vi "RH200 READ FILE.vi"() -> ()   [LabVIEW 2014]
uses:
  <vilib>/Utility/file.llb/Write To Spreadsheet File (string).vi
  <vilib>/DAQmx/write.llb/DAQmx Write (Analog DBL 1Chan 1Samp).vi
  <vilib>/DAQmx/write.llb/DAQmx Write (Digital Bool 1Line 1Point).vi
  <vilib>/DAQmx/read.llb/DAQmx Read (Analog DBL 1Chan 1Samp).vi
panel:
  in  "RH file":path
  out "Data file":path
  in  "Delay (s)":dbl=2.0 caption="Wet MFC (V)" format="%#_13g"
  in  "Log data":bool
  out "Saving data":bool
  in  "stop":bool
  out "Waveform Chart":cluster{"RH Setpoint":dbl, "RH":dbl}(graph)
  in  "Temp":dbl=25.0 caption="Temp (C)" format="%#_13g"
  # "REBOOT RH GENERATOR BETWEEN USES TO RESET CONNECTION TO PC"
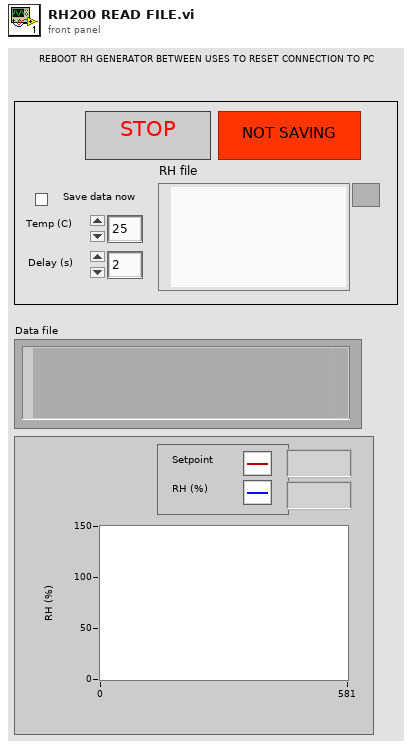
[diagram p1: front panel]
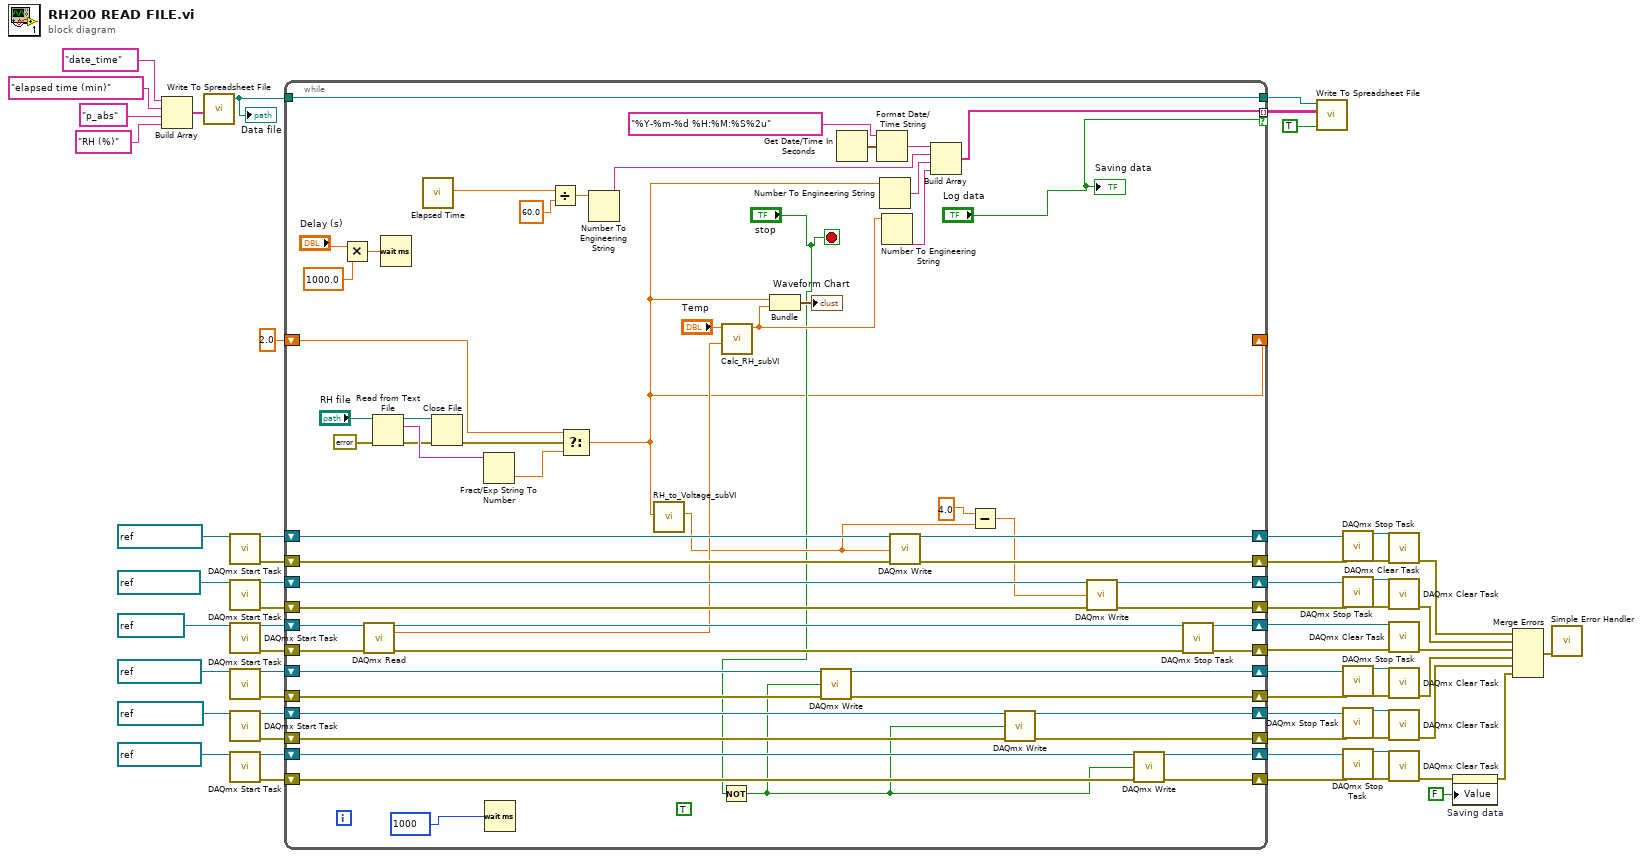
[diagram p0: block diagram]
diagram:
  n1 = Build Array("date_time" ("time format string (%c)"), "elapsed time (min)" ("time format string (%c)"), "p_abs" ("time format string (%c)"), "RH (%)" ("time format string (%c)")) -> (w9:string[])
  n2 = call-poly <vilib>:"Write To Spreadsheet File.vi"("1D data"=w9) -> ("new file path (Not A Path if cancelled)"=w11:path)  [unwired: 7 in]
  "Data file" <- w11
  n3 = call <vilib>:"DAQmx Start Task.vi"("task/channels in"=refnum<k21> "AO WET") -> ("task out"=w25:refnum<k21>, "error out"=w26:errorcluster)  [unwired: 13 in]
  n4 = call <vilib>:"DAQmx Start Task.vi"("task/channels in"=refnum<k21> "AO DRY") -> ("task out"=w28:refnum<k21>, "error out"=w27:errorcluster)  [unwired: 13 in]
  n5 = call <vilib>:"DAQmx Start Task.vi"("task/channels in"=refnum<k21> "AI DP") -> ("task out"=w58:refnum<k21>, "error out"=w57:errorcluster)  [unwired: 13 in]
  n6 = call <vilib>:"DAQmx Start Task.vi"("task/channels in"=refnum<k21> "DO DRY") -> ("task out"=w53:refnum<k21>, "error out"=w54:errorcluster)  [unwired: 13 in]
  n7 = call <vilib>:"DAQmx Start Task.vi"("task/channels in"=refnum<k21> "DO WET") -> ("task out"=w42:refnum<k21>, "error out"=w41:errorcluster)  [unwired: 13 in]
  n8 = call <vilib>:"DAQmx Start Task.vi"("task/channels in"=refnum<k21> "DO GAS") -> ("task out"=w39:refnum<k21>, "error out"=w40:errorcluster)  [unwired: 13 in]
  n9 = while {
    shift-right: [w112] -> w56
    shift-left: w58 -> [w119]
    shift-right: [w111] -> w55
    shift-left: w57 -> [w118]
    shift-right: [w108] -> w51
    shift-left: w53 -> [w109]
    shift-right: [w107] -> w48
    shift-left: w54 -> [w110]
    shift-right: [w105] -> w44
    shift-left: w42 -> [w104]
    shift-right: [w106] -> w47
    shift-left: w41 -> [w103]
    shift-right: [w100] -> w37
    shift-left: w39 -> [w101]
    shift-right: [w99] -> w34
    shift-left: w40 -> [w102]
    shift-right: [w97] -> w30
    shift-left: w28 -> [w96]
    shift-right: [w98] -> w33
    shift-left: w27 -> [w95]
    shift-right: [w92] -> w23
    shift-left: w25 -> [w93]
    shift-right: [w91] -> w20
    shift-left: w26 -> [w94]
    tunnel: [w90] -> w12
    tunnel: w11 -> [w90]
    tunnel: [w82] -> w7 mode=indexing if="Log data"
    shift-right: [w61] -> _
    shift-left: 2.0 -> [w63]
    stop <- "stop" stop-if-true
    (unwired) TRUE ("enable generator")
    n10 = Multiply(x="Delay (s)", y=1000.0) -> (x*y=w76:dbl)
    n11 = call-poly <vilib>:"DAQmx Read.vi"("task/channels in"=w119, "error in"=w118) -> ("task out"=w114:refnum<k21>, "data"=w73:dbl, "error out"=w113:errorcluster)  [unwired: 11 in]
    n12 = Read from Text File(file (use dialog)="RH file", error in=errorcluster {"status"=FALSE, "code"=0, "source"=""}) -> (refnum out=w66:refnum<file>, text=w67:string, error out=w65:errorcluster)  [unwired: 2 in, 1 out]
    n13 = Wait (ms)(milliseconds to wait=w76) -> ()  [unwired: 1 out]
    n14 = call "Elapsed Time"() -> ("Elapsed Time (s)"=w89:dbl)  [unwired: 12 in, 7 out]
    n15 = Close File(refnum=w66, error in=w65) -> (error out=w64:errorcluster)  [unwired: 1 out]
    n16 = Fract/Exp String To Number(string=w67) -> (number=w60:dbl)  [unwired: 3 in, 1 out]
    n17 = Wait (ms)(milliseconds to wait=u32 1000) -> ()  [unwired: 1 out]
    n18 = Divide(x=w89, y=60.0) -> (x/y=w84:dbl)
    n19 = Select(t=w63, s=w64, f=w60) -> (s? t:f=w61:dbl)
    n20 = Number To Engineering String ("elapsed time (min)")(4:w84) -> (0:w83:string)  [unwired: 3 in]
    n21 = call "RH_to_Voltage_subVI.vi"("RH"=w61) -> ("set point (V)"=w72:dbl)  [unwired: 10 in]
    n22 = Not(x="stop") -> (.not. x?=w71:bool)
    n23 = call "Calc_RH_subVI.vi"("DP"=w73, "Temp"="Temp") -> ("RH"=w80:dbl)  [unwired: 9 in]
    n24 = Bundle(w61, "RH"=w80) -> (→"Waveform Chart":cluster{dbl, "RH":dbl})  [unwired: 1 in]
    n25 = call-poly <vilib>:"DAQmx Write.vi"("task/channels in"=w109, "data"=w71, "error in"=w110) -> ("task out"=w108:refnum<k21>, "error out"=w107:errorcluster)  [unwired: 10 in, 1 out]
    n26 = Get Date/Time In Seconds() -> (seconds since 1Jan1904=w87:timestamp)
    n27 = Format Date/Time String(time format string (%c)="%Y-%m-%d %H:%M:%S%2u", seconds (now)=w87) -> (date/time string=w85:string)  [unwired: 1 in]
    n28 = Number To Engineering String ("elapsed time (min)")(4:w61) -> (0:w81:string)  [unwired: 3 in]
    n29 = Number To Engineering String ("elapsed time (min)")(4:w80) -> (0:w79:string)  [unwired: 3 in]
    n30 = call-poly <vilib>:"DAQmx Write.vi"("task/channels in"=w93, "data"=w72, "error in"=w94) -> ("task out"=w92:refnum<k21>, "error out"=w91:errorcluster)  [unwired: 10 in, 1 out]
    n31 = Build Array(w85, w83, w81, w79) -> (w82:string[])
    n32 = Subtract(x=4.0 ("data"), y=w72) -> (x-y=w74:dbl)
    n33 = call-poly <vilib>:"DAQmx Write.vi"("task/channels in"=w104, "data"=w71, "error in"=w103) -> ("task out"=w105:refnum<k21>, "error out"=w106:errorcluster)  [unwired: 10 in, 1 out]
    n34 = call-poly <vilib>:"DAQmx Write.vi"("task/channels in"=w96, "data"=w74, "error in"=w95) -> ("task out"=w97:refnum<k21>, "error out"=w98:errorcluster)  [unwired: 10 in, 1 out]
    n35 = call-poly <vilib>:"DAQmx Write.vi"("task/channels in"=w101, "data"=w71, "error in"=w102) -> ("task out"=w100:refnum<k21>, "error out"=w99:errorcluster)  [unwired: 10 in, 1 out]
    n36 = call <vilib>:"DAQmx Stop Task.vi"("task/channels in"=w114, "error in"=w113) -> ("task out"=w112:refnum<k21>, "error out"=w111:errorcluster)  [unwired: 12 in]
    "Saving data" <- "Log data"
  }
  n37 = call-poly <vilib>:"Write To Spreadsheet File.vi"("append to file? (new file:F)"=TRUE, "2D data"=w7, "file path (dialog if empty)"=w12) -> ()  [unwired: 5 in, 1 out]
  n38 = call <vilib>:"DAQmx Stop Task.vi"("task/channels in"=w23, "error in"=w20) -> ("task out"=w22:refnum<k21>, "error out"=w21:errorcluster)  [unwired: 12 in]
  n39 = call <vilib>:"DAQmx Stop Task.vi"("task/channels in"=w30, "error in"=w33) -> ("task out"=w31:refnum<k21>, "error out"=w32:errorcluster)  [unwired: 12 in]
  n40 = call <vilib>:"DAQmx Stop Task.vi"("task/channels in"=w51, "error in"=w48) -> ("task out"=w50:refnum<k21>, "error out"=w49:errorcluster)  [unwired: 12 in]
  n41 = call <vilib>:"DAQmx Stop Task.vi"("task/channels in"=w44, "error in"=w47) -> ("task out"=w45:refnum<k21>, "error out"=w46:errorcluster)  [unwired: 12 in]
  n42 = call <vilib>:"DAQmx Stop Task.vi"("task/channels in"=w37, "error in"=w34) -> ("task out"=w36:refnum<k21>, "error out"=w35:errorcluster)  [unwired: 12 in]
  n43 = call <vilib>:"DAQmx Clear Task.vi"("task in"=w22, "error in"=w21) -> ("error out"=w19:errorcluster)  [unwired: 13 in]
  n44 = call <vilib>:"DAQmx Clear Task.vi"("task in"=w31, "error in"=w32) -> ("error out"=w18:errorcluster)  [unwired: 13 in]
  n45 = call <vilib>:"DAQmx Clear Task.vi"("task in"=w56, "error in"=w55) -> ("error out"=w16:errorcluster)  [unwired: 13 in]
  n46 = call <vilib>:"DAQmx Clear Task.vi"("task in"=w50, "error in"=w49) -> ("error out"=w15:errorcluster)  [unwired: 13 in]
  n47 = call <vilib>:"DAQmx Clear Task.vi"("task in"=w45, "error in"=w46) -> ("error out"=w14:errorcluster)  [unwired: 13 in]
  n48 = call <vilib>:"DAQmx Clear Task.vi"("task in"=w36, "error in"=w35) -> ("error out"=w3:errorcluster)  [unwired: 13 in]
  n49 = property on="Saving data" class="Bool (strict)"(error in=w3, "Value"=FALSE ("enable generator")) -> (error out=w2:errorcluster)  [unwired: 1 in, 1 out]
  n50 = Merge Errors(w19, w18, w16, w15, w14, w2) -> (w17:errorcluster)
  n51 = call <vilib>:"Simple Error Handler.vi"("error in (no error)"=w17) -> ()  [unwired: 4 in, 5 out]
